vi "SilasTestingThingy.vi"() -> ()   [LabVIEW 2020]
panel:
  out "Seen_Game_Pieces":T1(array[cluster])
  in  "piece?":enum16{"None", "Cube", "Cone"}(ring)
  in  "Gamepiece Y":dbl
  in  "Gamepiece X":dbl
  in  "Confidence":dbl
  in  "Y (in) [t0]":dbl
  in  "X (in) [t0]":dbl
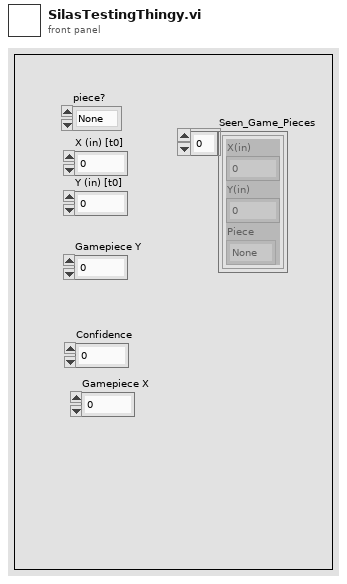
[diagram p1: front panel]
types:
  T1 = cluster{"X(in)":dbl, "Y(in)":dbl, "Piece":enum16{"None", "Cube", "Cone"}}[]
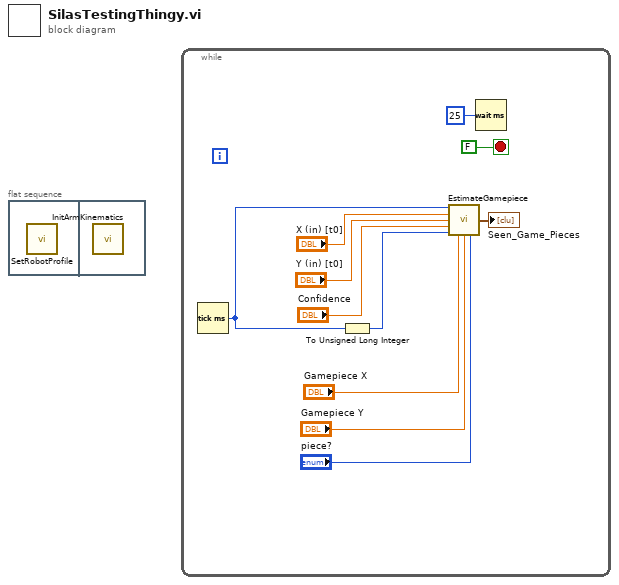
[diagram p0: block diagram]
diagram:
  n1 = flat-sequence {
    frame #0 {
      n2 = call "SetRobotProfile.vi"() -> ()  [unwired: 1 in]
    }
    frame #1 {
      n3 = call "InitArmKinematics.vi"() -> ()  [unwired: 1 in]
    }
  }
  n4 = while {
    stop <- FALSE stop-if-true
    n5 = Tick Count (ms)() -> (millisecond timer value=w3:u32)
    n6 = To Unsigned Long Integer(number=w3) -> (unsigned 32bit integer=w4:u32)
    n7 = call "EstimateGamepiece.vi"("Odometry Timestamp (ms)"=w3, "X (in) [t0]"="X (in) [t0]", "Y (in) [t0]"="Y (in) [t0]", "Confidence"="Confidence", "Vision Timestamp (ms)"=w4, "Gamepiece X"="Gamepiece X", "Gamepiece Y"="Gamepiece Y", "piece?"="piece?") -> ("Seen_Game_Pieces"=→"Seen_Game_Pieces":T1)  [unwired: 7 in]
    n8 = Wait (ms)(milliseconds to wait=u32 25) -> ()  [unwired: 1 out]
  }
